vi "엑셀 데이타 읽어오기.vi"(8 "열 길이":i32=3, 9 "행 길이":i32, 10 "시작 열":i32, 11 "시작 행":i32=205) -> (3 "배열":string[][](array[string]))   [LabVIEW 2015]
uses:
  <vilib>/addons/_office/excel.llb/Excel Get Data (str).vi
  <vilib>/Utility/NIReport.llb/NI_report.lvclass
  <vilib>/addons/_office/NI_ReportGenerationToolkit.lvlib
  <vilib>/Utility/NIReport.llb/Excel/NI_Excel.lvclass
panel:
  in  "start (0, 0)":cluster{"start row":i32, "start column":i32}
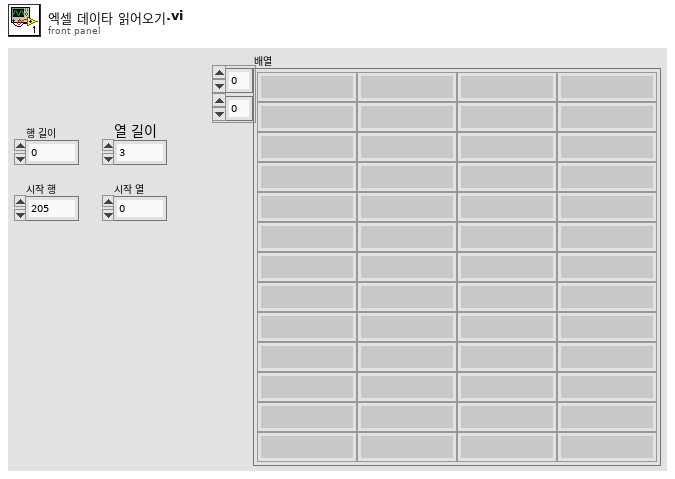
[diagram p1: front panel]
types:
  T1 = enum16{"Standard Report", "HTML", "Word", "Excel"}
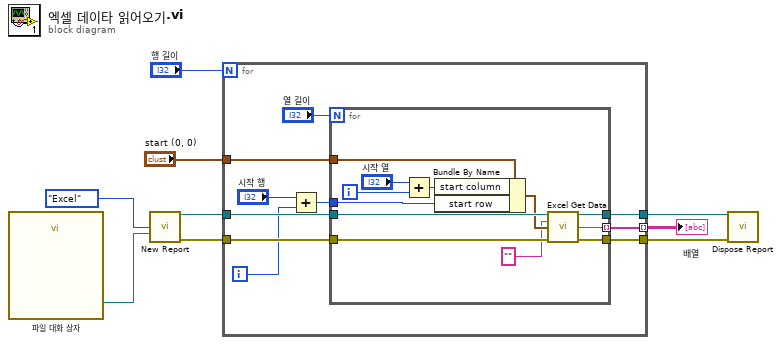
[diagram p0: block diagram]
diagram:
  n1 = call "파일 대화 상자"() -> ("selected path"=w9:path)  [unwired: 12 in, 3 out]
  n2 = call <vilib>:"New Report.vi"("report type"=T1."Excel", "template (empty)"=w9) -> ("report out"=w7:refnum<class "NI_report.lvclass">, "error out"=w8:errorcluster)  [unwired: 12 in]
  n3 = for {
    N: "행 길이" -> [_]
    tunnel: w8 -> [w19]
    tunnel: w7 -> [w18]
    tunnel: "start (0, 0)" -> [w17]
    tunnel: [w16] -> w3 mode=indexing
    tunnel: [w15] -> w4
    tunnel: [w14] -> w5
    i -> [w11]
    n4 = Add(x="시작 행", y=w11) -> (x+y=w12:i32)
    n5 = for {
      N: "열 길이" -> [_]
      tunnel: w19 -> [w31]
      tunnel: w18 -> [w30]
      tunnel: w17 -> [w29]
      tunnel: [w28] -> w16 mode=indexing
      tunnel: [w27] -> w15
      tunnel: [w26] -> w14
      tunnel: w12 -> [w22]
      i -> [w25]
      n6 = Add(x="시작 열", y=w25) -> (x+y=w21:i32)
      n7 = Bundle By Name(cluster=w29, "start column"=w21, "start row"=w22) -> (w24:cluster{"start row":i32, "start column":i32})
      n8 = call-poly <vilib>:"Excel Get Data.vi"("report in"=w30, "data type"="", "start (0, 0)"=w24, "error in (no error)"=w31) -> ("report out"=w26:refnum<class "NI_report.lvclass">, "data"=w28:string, "error out"=w27:errorcluster)  [unwired: 9 in]
    }
  }
  "배열" <- w3
  n9 = call-dynamic "Dispose Report.vi"("report in"=w5, "error in (no error)"=w4) -> ()  [unwired: 13 in, 1 out]
